vi "CUIT553_LOG_Ti_Ti_plus_driver.vi"(0 "DATA":string, 4 "error in (Log)":errorcluster, 5 "error in":T1) -> (15 "Ti float":string, 17 "Ti plus float":string)   [LabVIEW 2018]
uses:
  MOKO_LabViewLibrary/MokoLowLevel/MokoLowLovelControl/MLLC_Error.ctl
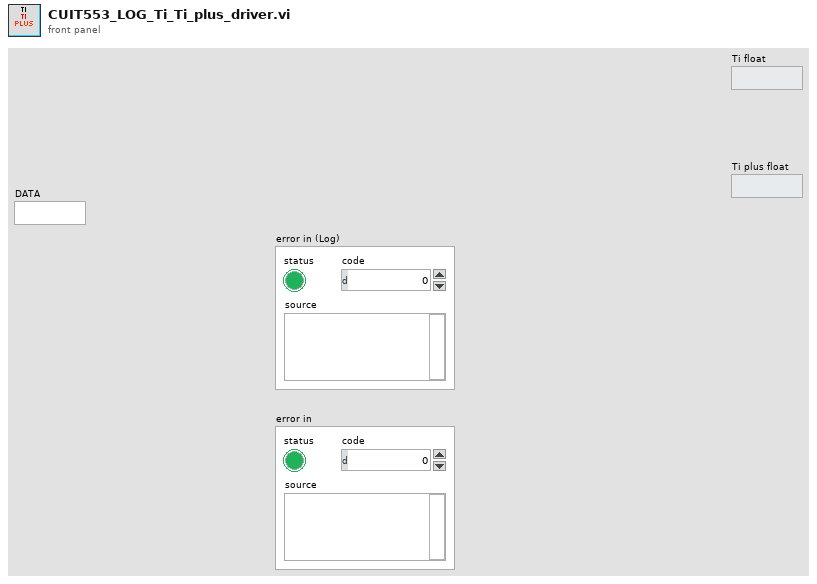
[diagram p1: front panel]
types:
  T1 = typedef "MLLC_Error.ctl" = errorcluster
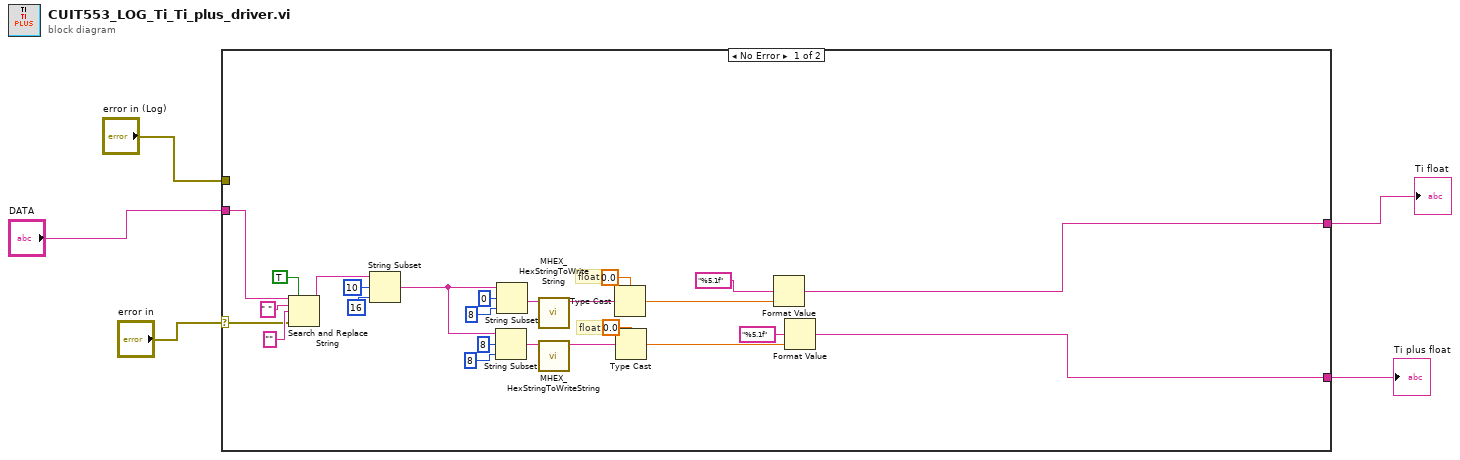
[diagram p0: block diagram]
diagram:
  n1 = case shown="No Error" "error in" {
    selector: "error in" -> [w27 _]
    tunnel: "DATA" -> [w22 _]
    tunnel: "error in (Log)" -> [_ _]
    tunnel: [w7 _] -> w4
    tunnel: [w6 _] -> w5
    frame No Error {
      # "float"
      # "float"
      n2 = Search and Replace String(replace all?=TRUE ("replace all? (F)"), input string=w22, search string=" ", replace string="" ("replace string (\"\")"), error in=w27) -> (result string=w25:string)  [unwired: 3 in, 3 out]
      n3 = String Subset(string=w25, offset (0)=10, length (rest)=16 ("length (rest)")) -> (substring=w23:string)
      n4 = String Subset(string=w23, offset (0)=8, length (rest)=8 ("length (rest)")) -> (substring=w13:string)
      n5 = String Subset(string=w23, offset (0)=0, length (rest)=8 ("length (rest)")) -> (substring=w15:string)
      n6 = call "MHEX_HexStringToWriteString.vi"("STRING HEX"=w15) -> ("String out"=w14:string)  [unwired: 7 in, 3 out]
      n7 = call "MHEX_HexStringToWriteString.vi"("STRING HEX"=w13) -> ("String out"=w12:string)  [unwired: 7 in, 3 out]
      n8 = Type Cast(type=sgl 0.0 ("32-bit IEEE 754"), x=w14) -> (*(type *) &x=w10:sgl)
      n9 = Type Cast(type=sgl 0.0 ("32-bit IEEE 754"), x=w12) -> (*(type *) &x=w8:sgl)
      n10 = Format Value(format string="%5.1f", value (0)=w10) -> (output string=w7:string)  [unwired: 1 in]
      n11 = Format Value(format string="%5.1f", value (0)=w8) -> (output string=w6:string)  [unwired: 1 in]
    }
    frame Error {
    }
  }
  "Ti plus float" <- w5
  "Ti float" <- w4
